vi "JAS_DashboardFormatCameraParams.vi"(10 "Camera Settings 2":T5, 11 "Camera Settings":T2={"name"="", "fps"=30, "compression"=30, "Image Size"=enum."320x240"}) -> (3 "parameter pairs":T6(array[cluster]))   [LabVIEW 2025]
uses:
  <vilib>/Rock Robotics/WPI/Camera/WPI_CameraExposure Values.ctl
  <vilib>/Rock Robotics/WPI/Camera/WPI_CameraWhite Balance Values.ctl
  JAS_CameraImageSize.ctl
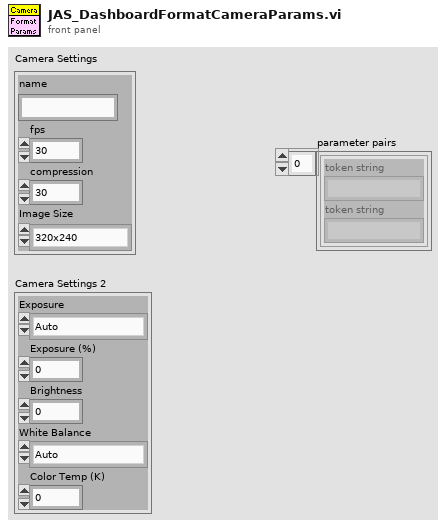
[diagram p1: front panel]
types:
  T1 = typedef "JAS_CameraImageSize.ctl" = enum16{"640x480", "640x360", "320x240", "320x180", "160x120", "160x90", "Custom"}
  T2 = cluster{"name":string, "fps":i32, "compression":i32, "Image Size":T1}
  T3 = typedef "WPI_CameraExposure Values.ctl" = enum16{"Auto", "Flicker-free 50 Hz", "Flicker-free 60 Hz", "Hold current", "Custom"}
  T4 = typedef "WPI_CameraWhite Balance Values.ctl" = enum16{"Auto", "Fixed indoor", "Fixed outdoor 1", "Fixed outdoor 2", "Fixed fluorescent 1", "Fixed fluorescent 2", "Hold current", "Custom"}
  T5 = cluster{"Exposure":T3, "Exposure (%)":dbl, "Brightness":i32, "White Balance":T4, "Color Temp (K)":dbl}
  T6 = cluster{"token string":string, "token string":string}[]
  T7 = cluster{"token string":string, "token string 2":string}[]
  T8 = cluster{"Exposure":bool, "Exposure (%)":bool, "Brightness":bool, "White Balance":bool, "Color Temp (K)":bool}
  T9 = cluster{"token string":string, "token string":string}
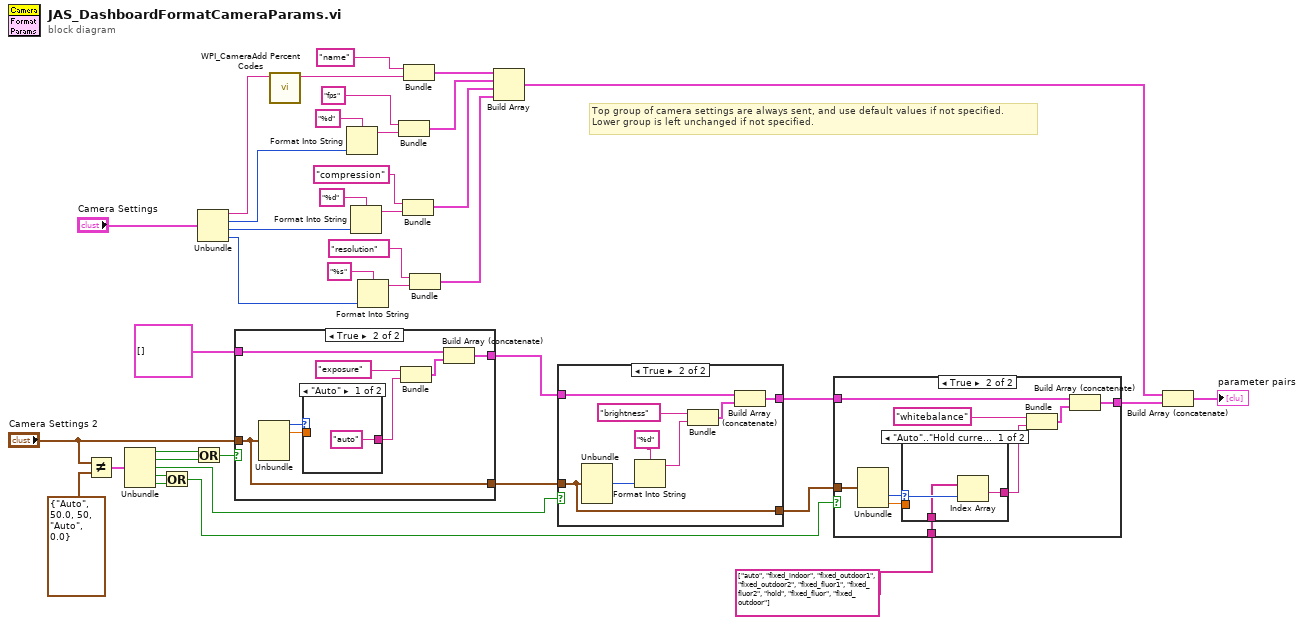
[diagram p0: block diagram]
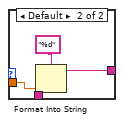
[diagram p3: hidden frame]
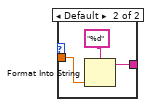
[diagram p6: hidden frame]
diagram:
  # "Top group of camera settings are always sent, and use default values if not specified.\nLower group is left unchanged if not specified."
  n1 = Not Equal?(x="Camera Settings 2", y=T5 {"Exposure"=enum."Auto", "Exposure (%)"=50.0, "Brightness"=50, "White Balance"=enum."Auto", "Color Temp (K)"=0.0} ("Camera Settings 2")) -> (x != y?=w24:T8)
  n2 = Unbundle(w24) -> ("Exposure"=w26:bool, "Exposure (%)"=w27:bool, "Brightness"=w37:bool, "White Balance"=w34:bool, "Color Temp (K)"=w35:bool)
  n3 = Or(x=w34, y=w35) -> (x .or. y?=w36:bool)
  n4 = Or(x=w26, y=w27) -> (x .or. y?=w25:bool)
  n5 = Unbundle("Camera Settings") -> ("name"=w23:string, "fps"=w10:i32, "compression"=w14:i32, "Image Size"=w21:T1)
  n6 = case shown="True" w25 {
    tunnel: "Camera Settings 2" -> [w40 w42]
    tunnel: T7 [] ("parameters") -> [w41 w45]
    tunnel: [w41 w44] -> w29
    tunnel: [w40 w42] -> w32
    frame False {
    }
    frame True {
      n7 = Unbundle(w42) -> ("Exposure"=w48:T3, "Exposure (%)"=w47:dbl)  [unwired: 3 out]
      n8 = case shown="\"Auto\"" w48 {
        tunnel: w47 -> [_ w53]
        tunnel: ["auto" ("token string") w52] -> w46
        frame "Auto" {
        }
        frame Default {
          n9 = Format Into String(format string="%d" ("token string"), w53) -> (resulting string=w52:string)  [unwired: 2 in, 1 out]
        }
      }
      n10 = Bundle("token string"="exposure", "token string"=w46) -> (w43:T9)  [unwired: 1 in]
      n11 = Build Array (concatenate)(w45, w43) -> (w44:T6)
    }
  }
  n12 = call <vilib>:"WPI_CameraAdd Percent Codes.vi"("String"=w23) -> ("String 2"=w8:string)  [unwired: 10 in]
  n13 = Format Into String(format string="%d", w10) -> (resulting string=w11:string)  [unwired: 2 in, 1 out]
  n14 = Format Into String(format string="%d", w14) -> (resulting string=w17:string)  [unwired: 2 in, 1 out]
  n15 = Format Into String(format string="%s", w21) -> (resulting string=w18:string)  [unwired: 2 in, 1 out]
  n16 = Bundle("fps", w11) -> (w6:cluster{string, string})  [unwired: 1 in]
  n17 = Bundle("compression", w17) -> (w5:cluster{string, string})  [unwired: 1 in]
  n18 = Bundle("name", "String 2"=w8) -> (w7:cluster{string, "String 2":string})  [unwired: 1 in]
  n19 = Bundle("resolution", w18) -> (w4:cluster{string, string})  [unwired: 1 in]
  n20 = Build Array(w7, w6, w5, w4) -> (w3:cluster{string, "String 2":string}[])
  n21 = case shown="True" w37 {
    tunnel: w32 -> [w54 w57]
    tunnel: w29 -> [w55 w61]
    tunnel: [w55 w60] -> w31
    tunnel: [w54 w57] -> w33
    frame False {
    }
    frame True {
      n22 = Unbundle(w57) -> ("Brightness"=w56:i32)  [unwired: 4 out]
      n23 = Format Into String(format string="%d" ("token string"), w56) -> (resulting string=w62:string)  [unwired: 2 in, 1 out]
      n24 = Bundle("token string"="brightness", w62) -> (w59:cluster{"token string":string, string})  [unwired: 1 in]
      n25 = Build Array (concatenate)(w61, w59) -> (w60:T6)
    }
  }
  n26 = case shown="True" w36 {
    tunnel: w33 -> [_ w72]
    tunnel: w31 -> [w64 w70]
    tunnel: [w64 w69] -> w2
    tunnel: string[] ["auto", "fixed_indoor", "fixed_outdoor1", "fixed_outdoor2", "fixed_fluor1", "fixed_fluor2", "hold", "fixed_fluor", "fixed_outdoor"] ("Array") -> [_ w65]
    frame False {
    }
    frame True {
      n27 = Unbundle(w72) -> ("White Balance"=w67:T4, "Color Temp (K)"=w66:dbl)  [unwired: 3 out]
      n28 = case shown="\"Auto\"..\"Hold current\"" w67 {
        selector: w67 -> [w76 _]
        tunnel: w66 -> [_ w79]
        tunnel: [w75 w78] -> w71
        tunnel: w65 -> [w74 _]
        frame "Auto".."Hold current" {
          n29 = Index Array(array=w74, index=w76) -> (element=w75:string)
        }
        frame Default {
          n30 = Format Into String(format string="%d" ("token string"), w79) -> (resulting string=w78:string)  [unwired: 2 in, 1 out]
        }
      }
      n31 = Bundle("token string"="whitebalance", w71) -> (w68:cluster{"token string":string, string})  [unwired: 1 in]
      n32 = Build Array (concatenate)(w70, w68) -> (w69:T6)
    }
  }
  n33 = Build Array (concatenate)(w3, w2) -> (→"parameter pairs":T6)
